vi "get control reference by name.vi"   [LabVIEW 2019]
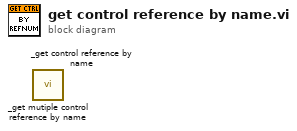
[diagram p0: block diagram]
diagram:
  n1 = call "_get mutiple control reference by name.vi"() -> ()  [unwired: 6 in, 2 out]
  n2 = call "_get control reference by name.vi"() -> ()  [unwired: 6 in, 2 out]
